vi "Aircraft 3 System Status.vi"(7 "Method":enum16{"Get", "Set"}(ring), 11 "System Status In":T1 {"Communication Drop Rate (%)" scale=0.0..100.0; "Battery Remaining (%)" scale=0.0..100.0; "CPU Load (%)" scale=0.0..100.0}) -> (3 "System Status Out":T1 {"Communication Drop Rate (%)" scale=0.0..100.0; "Battery Remaining (%)" scale=0.0..100.0; "CPU Load (%)" scale=0.0..100.0})   [LabVIEW 2014]
uses:
  Controls/Aircraft Sensor Status Data.ctl
  GUI Design/Indicators/Sensor Status LED CLuster.ctl
  GUI Design/Indicators/Status LED.ctl
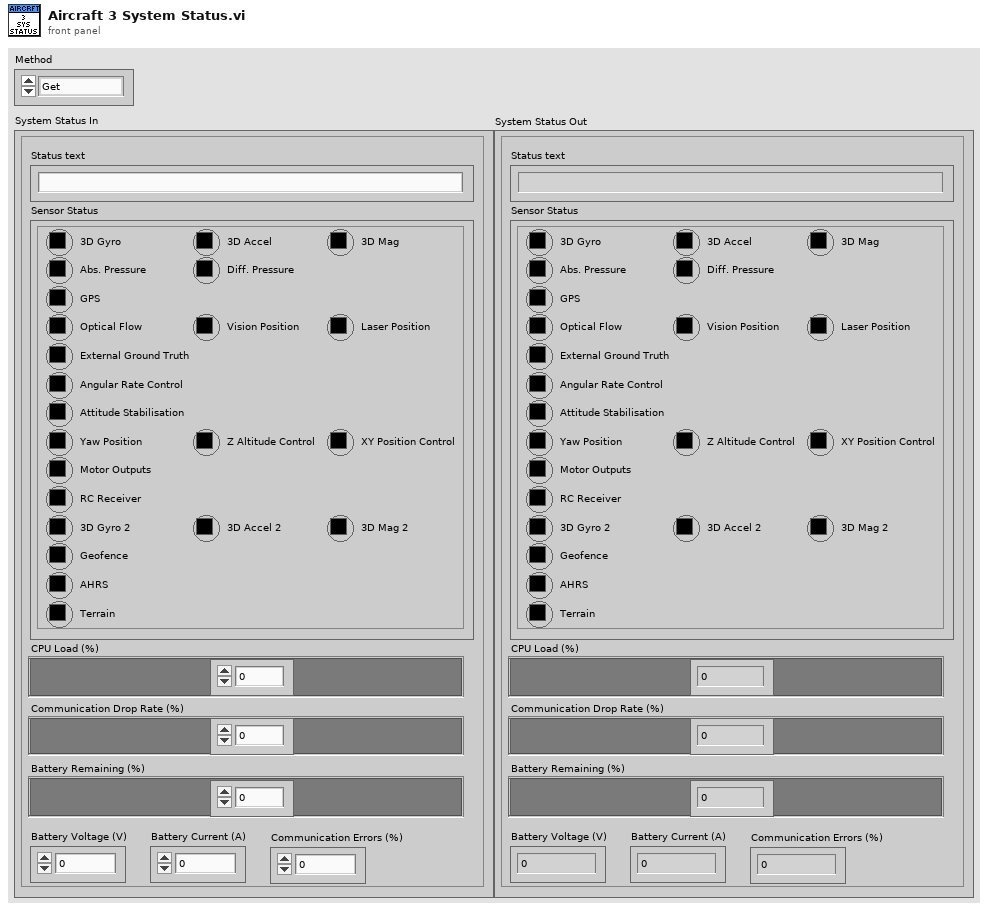
[diagram p1: front panel]
types:
  T1 = typedef "Aircraft Sensor Status Data.ctl" = cluster{"Sensor Status":T2, "CPU Load (%)":dbl, "Battery Voltage (V)":dbl, "Battery Current (A)":dbl, "Battery Remaining (%)":dbl, "Communication Drop Rate (%)":dbl, "Communication Errors (%)":dbl, "Status text":string}
  T2 = typedef "Sensor Status LED CLuster.ctl" = cluster{"3D Gyro":u32, "3D Accel":u32, "3D Mag":u32, "Abs. Pressure":u32, "Diff. Pressure":u32, "GPS":T3, "Optical Flow":u32, "Vision Position":u32, "Laser Position":u32, "External Ground Truth":u32, "Angular Rate Control":u32, "Attitude Stabilisation":u32, "Yaw Position":u32, "Z Altitude Control":u32, "XY Position Control":u32, "Motor Outputs":u32, "RC Receiver":u32, "3D Gyro 2":u32, "3D Accel 2":u32, "3D Mag 2":u32, "Geofence":u32, "AHRS":u32, "Terrain":u32}
  T3 = typedef "Status LED.ctl" = u32
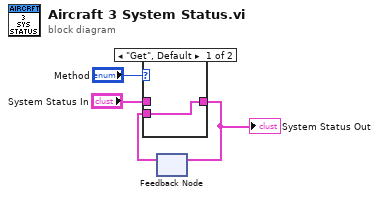
[diagram p0: block diagram]
diagram:
  n1 = feedback #1() -> (w1:T1)  [unwired: 1 in]
  n2 = case shown="\"Get\", Default" "Method" {
    tunnel: "System Status In" -> [_ w6]
    tunnel: [w5 w6] -> w2
    tunnel: w1 -> [w5 _]
    frame "Get", Default {
    }
    frame "Set" {
    }
  }
  "System Status Out" <- w2
  n3 = feedback-in #1(w2) -> ()
